vi "Channel Read.vi"(0 "Session Handle in":T3, 7 "ChannelSelection":T2, 11 "error in (no error)":errorcluster) -> (4 "Session Handle out":T3, 6 "Waveform Graph":dbl[](array[numeric]), 8 "[Meta]SetupInfoH":T1, 15 "error out":errorcluster)   [LabVIEW 2019, in "SmartScopeDriver.lvclass"]
uses:
  SmartScopeDriver.lvclass
  Typedefs/Session Handle.ctl
  Scope Driver/Typedef/Channel Selection.ctl
  Scope Driver/Typedef/Metadata/[Meta]SetupInfoH.ctl
  SmartScopeDriver.lvclass/SmartScopeDriver.ctl
  Scope Driver/LabNation Scope Driver.lvlib
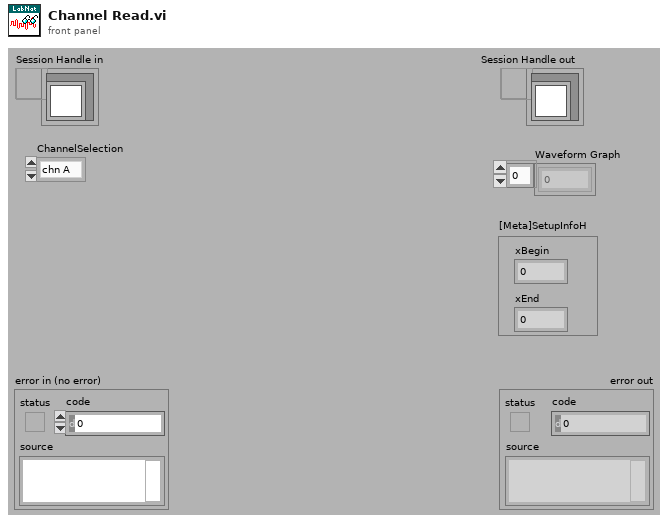
[diagram p1: front panel]
types:
  T1 = typedef "LabNation Scope Driver.lvlib/[Meta]SetupInfoH.ctl" = cluster{"xBegin":dbl, "xEnd":dbl}
  T2 = typedef "LabNation Scope Driver.lvlib/Channel Selection.ctl" = enum16{"chn A", "chn B"}
  T3 = typedef "SmartScopeDriver.lvclass/Session Handle.ctl" = refnum<data-value>
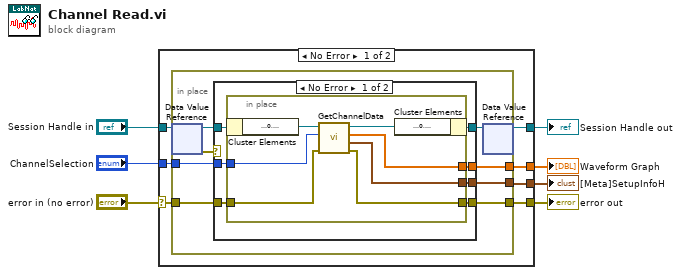
[diagram p0: block diagram]
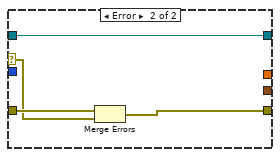
[diagram p2: hidden frame]
diagram:
  n1 = case shown="No Error" "error in (no error)" {
    selector: "error in (no error)" -> [w12 w41]
    tunnel: "Session Handle in" -> [w14 w42]
    tunnel: [w13 w42] -> w6
    tunnel: [w11 w41] -> w5
    tunnel: "ChannelSelection" -> [w10 _]
    tunnel: [w9 _] -> w2
    tunnel: [w8 _] -> w1
    frame No Error {
      n2 = in-place {
        in-place-border: w12 -> [w18]
        in-place-border: [w21] -> w11
        in-place-border: w10 -> [w17]
        in-place-border: [w16] -> w9
        in-place-border: [w15] -> w8
        n3 = in-place-dvr #1(w14) -> (w22:refnum<class "SmartScopeDriver.lvclass">, w19:errorcluster)
        n4 = case shown="No Error" w19 {
          selector: w19 -> [_ w39]
          tunnel: w22 -> [w29 w37]
          tunnel: [w28 w38] -> w21
          tunnel: [w27 w37] -> w20
          tunnel: w18 -> [w26 w40]
          tunnel: w17 -> [w25 _]
          tunnel: [w24 _] -> w16
          tunnel: [w23 _] -> w15
          frame No Error {
            n5 = in-place {
              in-place-border: [w35] -> w28
              in-place-border: w26 -> [w36]
              in-place-border: w25 -> [w32]
              in-place-border: [w31] -> w24
              in-place-border: [w30] -> w23
              n6 = in-place-cluster #2(w29) -> ("reference"=w34:refnum<k24>)
              n7 = call "GetChannelData.vi"("error in (no error)"=w36, "ChannelSelection"=w32, "reference in"=w34) -> ("error out"=w35:errorcluster, "[Meta]SetupInfoH"=w30:T1, "Waveform Graph"=w31:dbl[], "reference out"=w33:refnum<k24>)  [unwired: 5 in]
              n8 = in-place-cluster #2("reference"=w33) -> (w27:refnum<class "SmartScopeDriver.lvclass">)
            }
          }
          frame Error {
            n9 = Merge Errors(w40, w39) -> (w38:errorcluster)
          }
        }
        n10 = in-place-dvr #1(w20) -> (w13:T3)  [unwired: 1 out]
      }
    }
    frame Error {
    }
  }
  "Session Handle out" <- w6
  "error out" <- w5
  "[Meta]SetupInfoH" <- w1
  "Waveform Graph" <- w2
